vi "_Close Dead References.vi"(1 "VI Ref Array In":refnum<vi>[](array[refnum])) -> (0 "VI Ref Array Out":refnum<vi>[](array[refnum]))   [LabVIEW 2012]
doc: "_Drop Closed References.vi\n\nPurpose: The title is a little misleading. The VI takes an array of references, and closes all those whose front panels are closed. The array of references returned is equal to the original array, without the references that have now been closed."
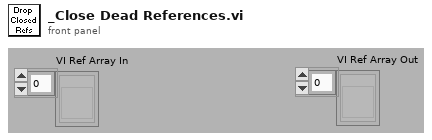
[diagram p1: front panel]
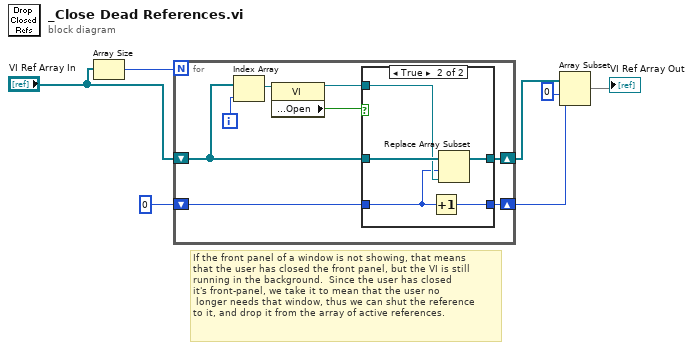
[diagram p0: block diagram]
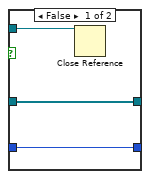
[diagram p2: hidden frame]
diagram:
  # "If the front panel of a window is not showing, that means\nthat the user has closed the front panel, but the VI is still\nrunning in the background.  Since the user has closed \nit's front-panel, we take it to mean that the user no\n longer needs that window, thus we can shut the reference\nto it, and drop it from the array of active references."
  n1 = Array Size(array="VI Ref Array In") -> (size(s)=w6:i32)
  n2 = for {
    N: w6 -> [_]
    shift-right: [w11] -> w3
    shift-left: 0 -> [w13]
    shift-right: [w12] -> w2
    shift-left: "VI Ref Array In" -> [w9]
    i -> [w14]
    n3 = Index Array(array=w9, index=w14) -> (element=w8:refnum<vi>)
    n4 = property class="VI"(reference=w8) -> (reference out=w15:refnum<vi>, "Front Panel Window:Open"=w10:bool)  [unwired: 1 in, 1 out]
    n5 = case shown="True" w10 {
      tunnel: w15 -> [w16 w22]
      tunnel: w9 -> [w18 w23]
      tunnel: w13 -> [w17 w20]
      tunnel: [w18 w21] -> w12
      tunnel: [w17 w19] -> w11
      frame False {
        n6 = Close Reference(reference=w16) -> ()  [unwired: 1 in, 1 out]
      }
      frame True {
        n7 = Increment(x=w20) -> (x+1=w19:i32)
        n8 = Replace Array Subset(array=w23, new element=w22, index=w20) -> (w21:refnum<vi>[])
      }
    }
  }
  n9 = Array Subset(array=w2, index=0, length=w3) -> (→"VI Ref Array Out":refnum<vi>[])
